vi "FTW-ScripterStep-Base_Timeout_Set.vi"(8 "error in (no error)":errorcluster, 10 "Timeout":dbl=-1.0 format="%<%H:%M:%S%3u>t", 11 "FTW-ScripterStep-Base In":refnum<class "FTW-ScripterStep-Base.lvclass">) -> (0 "error out":errorcluster, 3 "FTW-ScripterStep-Base Out":refnum<class "FTW-ScripterStep-Base.lvclass">)   [LabVIEW 2015, in "FTW-ScripterStep-Base.lvclass"]
uses:
  FTW-ScripterStep-Base.lvclass
  FTW-ScripterStep-Base.lvclass/FTW-ScripterStep-Base.ctl
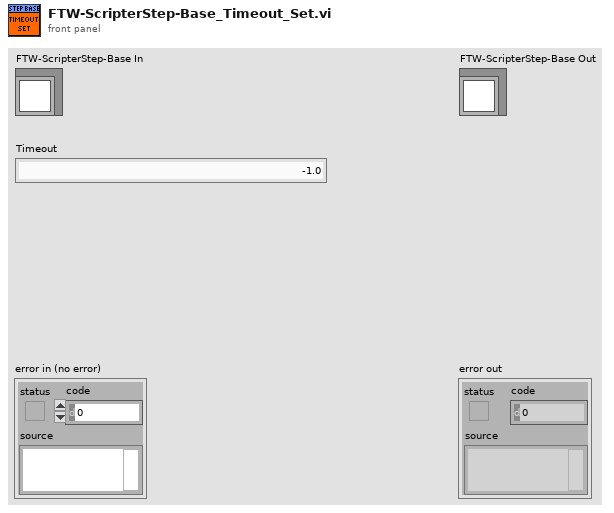
[diagram p1: front panel]
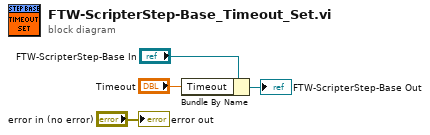
[diagram p0: block diagram]
diagram:
  n1 = Bundle By Name(cluster="FTW-ScripterStep-Base In", "Timeout"="Timeout") -> (→"FTW-ScripterStep-Base Out":refnum<class "FTW-ScripterStep-Base.lvclass">)
  "error out" <- "error in (no error)"
